vi "Leakdaten laden_speichern.vi"(6 "Aktion":T4(ring), 8 "error in (no error)":errorcluster caption="Fehler (Eingang, kein Fehler)", 9 "Leak Protokoll":T1={"Bearbeiter:"="", "Pfad:"=path "D:/IAG_Data/Log", "Textname:"="", "Analysator"=""} caption="T90 Konfig Daten", 11 "Gesamtvolumen":T3 {"LeakValve" items=["inactive", "active"]}) -> (0 "error out":errorcluster caption="Fehler (Ausgang)", 1 "Leak Protokoll":T1={"Bearbeiter:"="", "Pfad:"=path "D:/IAG_Data/Log", "Textname:"="", "Analysator"=""} caption="T90 Konfig Daten", 3 "Gesamtvolumen":T3 {"LeakValve" items=["inactive", "active"]})   [LabVIEW 2020, in "EPA 1065.lvlib" / "Dichtheitstest 1065-345.lvlib"]
uses:
  Dichtheitstest 1065-345.lvlib
  Gesamtvolumen.ctl
  Leak Protokoll Einstellungen.ctl
  Seiten/System Einstellungen V2/Analysatoren.ctl
  <vilib>/Utility/config.llb/Read Key (Double).vi
  <vilib>/Utility/config.llb/Read Key (Boolean).vi
  <vilib>/Utility/config.llb/Read Key (U32).vi
  <vilib>/Utility/config.llb/Write Key (Double).vi
  <vilib>/Utility/config.llb/Write Key (Boolean).vi
  <vilib>/Utility/config.llb/Write Key (U32).vi
  <vilib>/Utility/config.llb/Read Key (Path).vi
  <vilib>/Utility/config.llb/Read Key (String).vi
  <vilib>/Utility/config.llb/Write Key (Path).vi
  <vilib>/Utility/config.llb/Write Key (String).vi
  <vilib>/Utility/config.llb/NI_LVConfig.lvlib
  Allgemein/allgemeine Sub-VIs.lvlib
  Seiten/System Einstellungen V2/System Einstellungen V2.lvlib
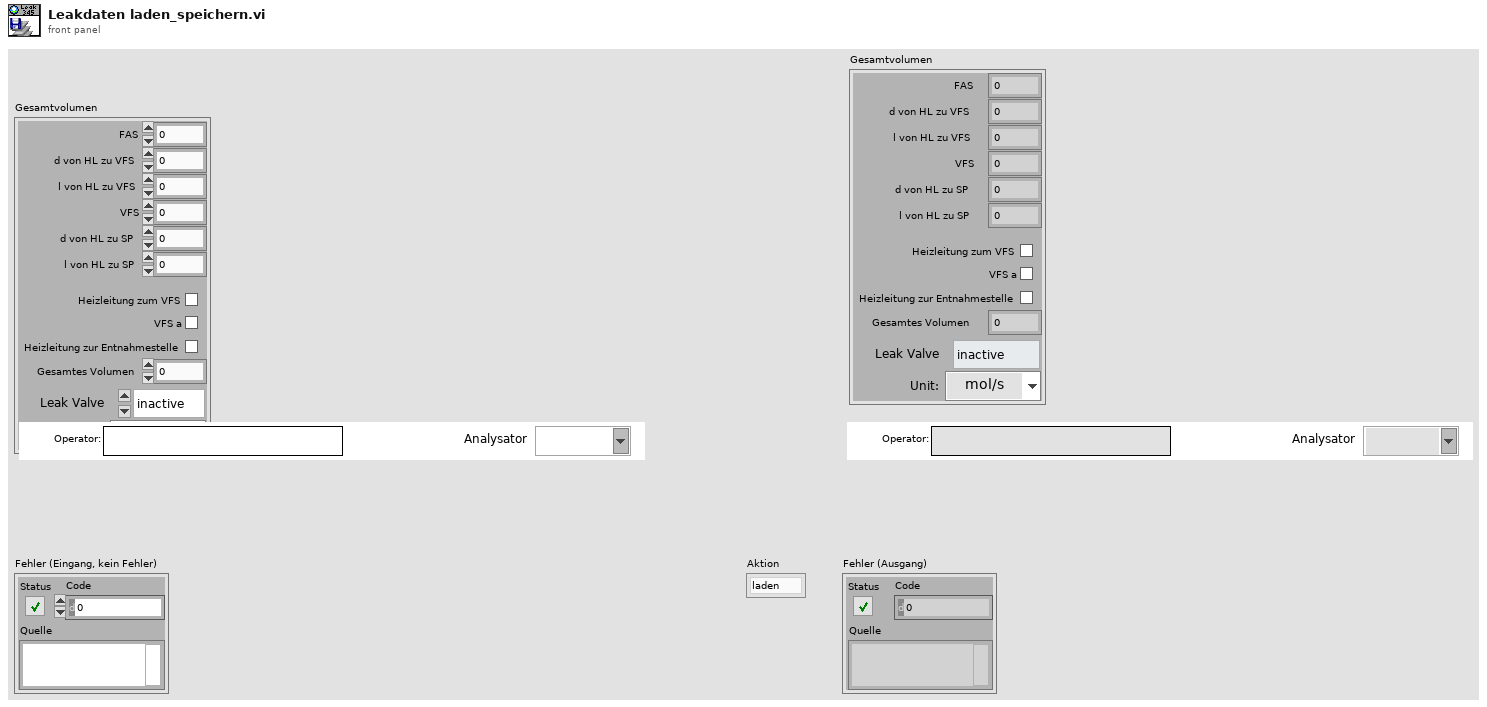
[diagram p1: front panel]
types:
  T1 = typedef "EPA 1065.lvlib/Dichtheitstest 1065-345.lvlib/Leak Protokoll Einstellungen.ctl" = cluster{"Bearbeiter:":string, "Pfad:":path, "Textname:":string, "Analysator":T2}
  T2 = typedef "System Einstellungen V2.lvlib/Analysatoren.ctl" = string
  T3 = typedef "EPA 1065.lvlib/Dichtheitstest 1065-345.lvlib/Gesamtvolumen.ctl" = cluster{"FAS":sgl, "d von HL zu VFS":sgl, "l von HL zu VFS":sgl, "VFS":sgl, "d von HL zu SP":sgl, "l von HL zu SP":sgl, "Heizleitung zum VFS":bool, "VFS a":bool, "Heizleitung zur Entnahmestelle":bool, "Gesamtes Volumen":sgl, "LeakValve":u16, "Einheit":enum16{"mol/s", "mbar"}}
  T4 = enum16{"laden", "speichern", "Pfad laden", "Pfad speichern"}
  T5 = typedef "NI_LVConfig.lvlib/Config Data RefNum.ctl" = refnum<k1>
  T6 = cluster{sgl, sgl, sgl, sgl, sgl, sgl, "value":bool, "value":bool, "value":bool, sgl, u16, u16}
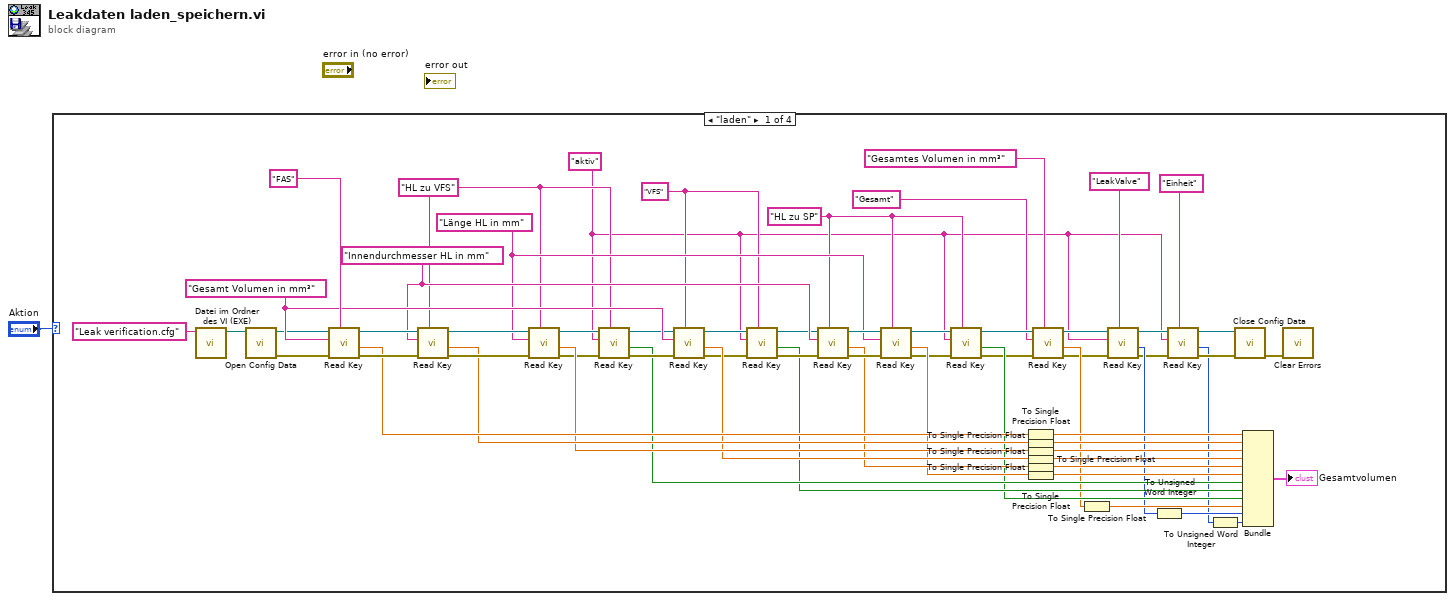
[diagram p0: block diagram]
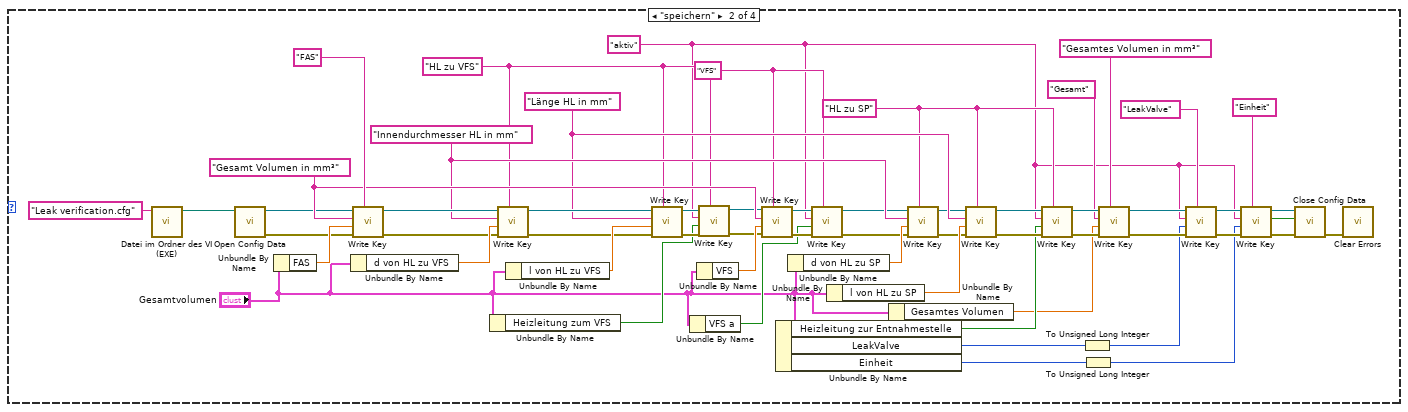
[diagram p2: hidden frame]
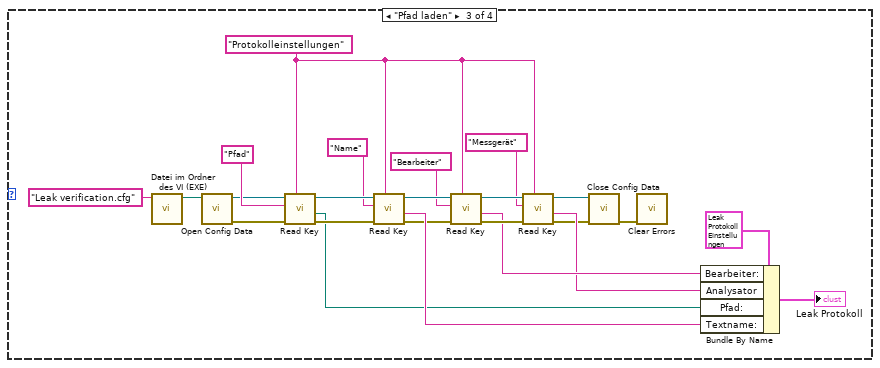
[diagram p3: hidden frame]
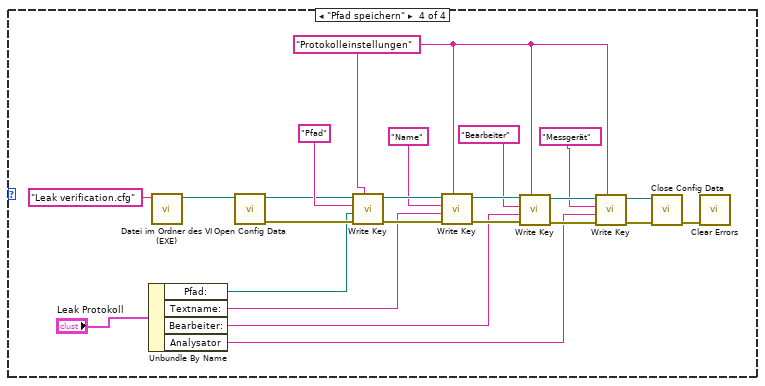
[diagram p4: hidden frame]
diagram:
  n1 = case shown="\"laden\"" "Aktion" {
    frame "laden" {
      w4 = "aktiv" ("key")
      w33 = "VFS"
      w29 = "HL zu SP"
      w55 = "Länge HL in mm" ("key")
      w56 = "Innendurchmesser HL in mm" ("key")
      w41 = "HL zu VFS"
      w57 = "Gesamt Volumen in mm³" ("key")
      n2 = call "Datei im Ordner des VI (EXE).vi"("Dateiname"="Leak verification.cfg") -> ("Dateipfad im Ordner des Haupt-VIs"=w51:path)  [unwired: 8 in, 2 out]
      n3 = call <vilib>:"Open Config Data.vi"("configuration file path"=w51) -> ("error out"=w53:errorcluster, "refnum"=w52:T5)  [unwired: 8 in, 1 out]
      n4 = call-poly <vilib>:"Read Key.vi"("section"="FAS", "error in (no error)"=w53, "key"=w57, "refnum"=w52) -> ("error out"=w61:errorcluster, "value"=w49:dbl, "refnum out"=w62:T5)  [unwired: 4 in, 1 out]
      n5 = call-poly <vilib>:"Read Key.vi"("section"=w41, "error in (no error)"=w61, "key"=w56, "refnum"=w62) -> ("error out"=w59:errorcluster, "value"=w48:dbl, "refnum out"=w63:T5)  [unwired: 4 in, 1 out]
      n6 = call-poly <vilib>:"Read Key.vi"("section"=w41, "error in (no error)"=w59, "key"=w55, "refnum"=w63) -> ("error out"=w40:errorcluster, "value"=w47:dbl, "refnum out"=w43:T5)  [unwired: 4 in, 1 out]
      n7 = call-poly <vilib>:"Read Key.vi"("section"=w41, "error in (no error)"=w40, "key"=w4, "refnum"=w43) -> ("error out"=w39:errorcluster, "value"=w38:bool, "refnum out"=w42:T5)  [unwired: 4 in, 1 out]
      n8 = call-poly <vilib>:"Read Key.vi"("section"=w33, "error in (no error)"=w39, "key"=w57, "refnum"=w42) -> ("error out"=w36:errorcluster, "value"=w46:dbl, "refnum out"=w37:T5)  [unwired: 4 in, 1 out]
      n9 = call-poly <vilib>:"Read Key.vi"("section"=w33, "error in (no error)"=w36, "key"=w4, "refnum"=w37) -> ("error out"=w35:errorcluster, "value"=w32:bool, "refnum out"=w34:T5)  [unwired: 4 in, 1 out]
      n10 = call-poly <vilib>:"Read Key.vi"("section"=w29, "error in (no error)"=w35, "key"=w56, "refnum"=w34) -> ("error out"=w58:errorcluster, "value"=w45:dbl, "refnum out"=w60:T5)  [unwired: 4 in, 1 out]
      n11 = call-poly <vilib>:"Read Key.vi"("section"=w29, "error in (no error)"=w58, "key"=w55, "refnum"=w60) -> ("error out"=w30:errorcluster, "value"=w44:dbl, "refnum out"=w31:T5)  [unwired: 4 in, 1 out]
      n12 = call-poly <vilib>:"Read Key.vi"("section"=w29, "error in (no error)"=w30, "key"=w4, "refnum"=w31) -> ("error out"=w19:errorcluster, "value"=w28:bool, "refnum out"=w18:T5)  [unwired: 4 in, 1 out]
      n13 = To Single Precision Float(number=w49) -> (single precision float=w26:sgl)
      n14 = To Single Precision Float(number=w48) -> (single precision float=w25:sgl)
      n15 = To Single Precision Float(number=w47) -> (single precision float=w24:sgl)
      n16 = To Single Precision Float(number=w46) -> (single precision float=w23:sgl)
      n17 = To Single Precision Float(number=w45) -> (single precision float=w22:sgl)
      n18 = To Single Precision Float(number=w44) -> (single precision float=w21:sgl)
      n19 = call-poly <vilib>:"Read Key.vi"("section"="Gesamtes Volumen in mm³", "error in (no error)"=w19, "key"="Gesamt", "refnum"=w18) -> ("error out"=w13:errorcluster, "value"=w17:dbl, "refnum out"=w14:T5)  [unwired: 4 in, 1 out]
      n20 = To Single Precision Float(number=w17) -> (single precision float=w20:sgl)
      n21 = call-poly <vilib>:"Read Key.vi"("section"="LeakValve", "error in (no error)"=w13, "key"=w4, "refnum"=w14) -> ("error out"=w9:errorcluster, "value"=w10:u32, "refnum out"=w8:T5)  [unwired: 4 in, 1 out]
      n22 = To Unsigned Word Integer(number=w10) -> (unsigned 16bit integer=w11:u16)
      n23 = call-poly <vilib>:"Read Key.vi"("section"="Einheit" ("key"), "error in (no error)"=w9, "key"=w4, "refnum"=w8) -> ("error out"=w6:errorcluster, "value"=w3:u32, "refnum out"=w7:T5)  [unwired: 4 in, 1 out]
      n24 = To Unsigned Word Integer(number=w3) -> (unsigned 16bit integer=w2:u16)
      n25 = call <vilib>:"Close Config Data.vi"("error in (no error)"=w6, "refnum"=w7) -> ("error out"=w54:errorcluster)  [unwired: 8 in, 1 out]
      n26 = Bundle(w26, w25, w24, w23, w22, w21, "value"=w38, "value"=w32, "value"=w28, w20, w11, w2) -> (→"Gesamtvolumen":T6)  [unwired: 1 in]
      n27 = call <vilib>:"Clear Errors.vi"("error in (no error)"=w54) -> ()  [unwired: 5 in, 2 out]
    }
    frame "speichern" {
      w69 = "aktiv" ("key")
      w92 = "VFS"
      w86 = "HL zu SP"
      w108 = "Länge HL in mm" ("key")
      w109 = "Innendurchmesser HL in mm" ("key")
      w97 = "HL zu VFS"
      w110 = "Gesamt Volumen in mm³" ("key")
      n28 = call "Datei im Ordner des VI (EXE).vi"("Dateiname"="Leak verification.cfg") -> ("Dateipfad im Ordner des Haupt-VIs"=w104:path)  [unwired: 8 in, 2 out]
      n29 = call <vilib>:"Open Config Data.vi"("configuration file path"=w104) -> ("error out"=w106:errorcluster, "refnum"=w105:T5)  [unwired: 8 in, 1 out]
      n30 = Unbundle By Name("Gesamtvolumen") -> ("FAS"=w120:sgl)
      n31 = Unbundle By Name("Gesamtvolumen") -> ("d von HL zu VFS"=w119:sgl)
      n32 = call-poly <vilib>:"Write Key.vi"("section"="FAS", "error in (no error)"=w106, "value"=w120, "key"=w110, "refnum"=w105) -> ("error out"=w115:errorcluster, "refnum out"=w116:T5)  [unwired: 4 in, 1 out]
      n33 = Unbundle By Name("Gesamtvolumen") -> ("Heizleitung zum VFS"=w98:bool)
      n34 = call-poly <vilib>:"Write Key.vi"("section"=w97, "error in (no error)"=w115, "value"=w119, "key"=w109, "refnum"=w116) -> ("error out"=w111:errorcluster, "refnum out"=w117:T5)  [unwired: 4 in, 1 out]
      n35 = Unbundle By Name("Gesamtvolumen") -> ("l von HL zu VFS"=w118:sgl)
      n36 = call-poly <vilib>:"Write Key.vi"("section"=w97, "error in (no error)"=w111, "value"=w118, "key"=w108, "refnum"=w117) -> ("error out"=w102:errorcluster, "refnum out"=w101:T5)  [unwired: 4 in, 1 out]
      n37 = Unbundle By Name("Gesamtvolumen") -> ("VFS a"=w91:bool)
      n38 = Unbundle By Name("Gesamtvolumen") -> ("VFS"=w112:sgl)
      n39 = call-poly <vilib>:"Write Key.vi"("section"=w97, "error in (no error)"=w102, "value"=w98, "key"=w69, "refnum"=w101) -> ("error out"=w99:errorcluster, "refnum out"=w100:T5)  [unwired: 4 in, 1 out]
      n40 = call-poly <vilib>:"Write Key.vi"("section"=w92, "error in (no error)"=w99, "value"=w112, "key"=w110, "refnum"=w100) -> ("error out"=w96:errorcluster, "refnum out"=w95:T5)  [unwired: 4 in, 1 out]
      n41 = Unbundle By Name("Gesamtvolumen") -> ("Heizleitung zur Entnahmestelle"=w85:bool, "LeakValve"=w68:u16, "Einheit"=w66:enum16{"mol/s", "mbar"})
      n42 = Unbundle By Name("Gesamtvolumen") -> ("d von HL zu SP"=w113:sgl)
      n43 = call-poly <vilib>:"Write Key.vi"("section"=w92, "error in (no error)"=w96, "value"=w91, "key"=w69, "refnum"=w95) -> ("error out"=w93:errorcluster, "refnum out"=w94:T5)  [unwired: 4 in, 1 out]
      n44 = Unbundle By Name("Gesamtvolumen") -> ("l von HL zu SP"=w114:sgl)
      n45 = Unbundle By Name("Gesamtvolumen") -> ("Gesamtes Volumen"=w79:sgl)
      n46 = call-poly <vilib>:"Write Key.vi"("section"=w86, "error in (no error)"=w93, "value"=w113, "key"=w109, "refnum"=w94) -> ("error out"=w89:errorcluster, "refnum out"=w90:T5)  [unwired: 4 in, 1 out]
      n47 = call-poly <vilib>:"Write Key.vi"("section"=w86, "error in (no error)"=w89, "value"=w114, "key"=w108, "refnum"=w90) -> ("error out"=w88:errorcluster, "refnum out"=w87:T5)  [unwired: 4 in, 1 out]
      n48 = call-poly <vilib>:"Write Key.vi"("section"=w86, "error in (no error)"=w88, "value"=w85, "key"=w69, "refnum"=w87) -> ("error out"=w84:errorcluster, "refnum out"=w83:T5)  [unwired: 4 in, 1 out]
      n49 = To Unsigned Long Integer(number=w68) -> (unsigned 32bit integer=w67:u32)
      n50 = To Unsigned Long Integer(number=w66) -> (unsigned 32bit integer=w65:u32)
      n51 = call-poly <vilib>:"Write Key.vi"("section"="Gesamtes Volumen in mm³", "error in (no error)"=w84, "value"=w79, "key"="Gesamt", "refnum"=w83) -> ("error out"=w73:errorcluster, "refnum out"=w78:T5)  [unwired: 4 in, 1 out]
      n52 = call-poly <vilib>:"Write Key.vi"("section"="LeakValve", "error in (no error)"=w73, "value"=w67, "key"=w69, "refnum"=w78) -> ("error out"=w72:errorcluster, "refnum out"=w75:T5)  [unwired: 4 in, 1 out]
      n53 = call-poly <vilib>:"Write Key.vi"("section"="Einheit", "error in (no error)"=w72, "value"=w65, "key"=w69, "refnum"=w75) -> ("error out"=w71:errorcluster, "found?"=w76:bool, "refnum out"=w74:T5)  [unwired: 4 in]
      n54 = call <vilib>:"Close Config Data.vi"("error in (no error)"=w71, "write file if changed (T)"=w76, "refnum"=w74) -> ("error out"=w107:errorcluster)  [unwired: 7 in, 1 out]
      n55 = call <vilib>:"Clear Errors.vi"("error in (no error)"=w107) -> ()  [unwired: 5 in, 2 out]
    }
    frame "Pfad laden" {
      w126 = "Protokolleinstellungen"
      n56 = call "Datei im Ordner des VI (EXE).vi"("Dateiname"="Leak verification.cfg") -> ("Dateipfad im Ordner des Haupt-VIs"=w138:path)  [unwired: 8 in, 2 out]
      n57 = call <vilib>:"Open Config Data.vi"("configuration file path"=w138) -> ("error out"=w140:errorcluster, "refnum"=w139:T5)  [unwired: 8 in, 1 out]
      n58 = call-poly <vilib>:"Read Key.vi"("section"=w126, "error in (no error)"=w140, "key"="Pfad", "refnum"=w139) -> ("error out"=w144:errorcluster, "value"=w134:path, "refnum out"=w145:T5)  [unwired: 4 in, 1 out]
      n59 = call-poly <vilib>:"Read Key.vi"("section"=w126, "error in (no error)"=w144, "key"="Name", "refnum"=w145) -> ("error out"=w131:errorcluster, "value"=w135:string, "refnum out"=w132:T5)  [unwired: 4 in, 1 out]
      n60 = call-poly <vilib>:"Read Key.vi"("section"=w126, "error in (no error)"=w131, "key"="Bearbeiter", "refnum"=w132) -> ("error out"=w130:errorcluster, "value"=w125:string, "refnum out"=w129:T5)  [unwired: 4 in, 1 out]
      n61 = call-poly <vilib>:"Read Key.vi"("section"=w126, "error in (no error)"=w130, "key"="Messgerät", "refnum"=w129) -> ("error out"=w123:errorcluster, "value"=w124:string, "refnum out"=w122:T5)  [unwired: 4 in, 1 out]
      n62 = call <vilib>:"Close Config Data.vi"("error in (no error)"=w123, "refnum"=w122) -> ("error out"=w141:errorcluster)  [unwired: 8 in, 1 out]
      n63 = call <vilib>:"Clear Errors.vi"("error in (no error)"=w141) -> ()  [unwired: 5 in, 2 out]
      n64 = Bundle By Name(cluster=T1 {"Bearbeiter:"="", "Pfad:"=path "D:/IAG_Data/Log", "Textname:"="", "Analysator"=""} ("Leak Protokoll"), "Bearbeiter:"=w125, "Analysator"=w124, "Pfad:"=w134, "Textname:"=w135) -> (→"Leak Protokoll":T1)
    }
    frame "Pfad speichern" {
      w147 = "Protokolleinstellungen"
      n65 = Unbundle By Name("Leak Protokoll") -> ("Pfad:"=w158:path, "Textname:"=w157:string, "Bearbeiter:"=w152:string, "Analysator"=w146:T2)
      n66 = call "Datei im Ordner des VI (EXE).vi"("Dateiname"="Leak verification.cfg") -> ("Dateipfad im Ordner des Haupt-VIs"=w161:path)  [unwired: 8 in, 2 out]
      n67 = call <vilib>:"Open Config Data.vi"("configuration file path"=w161) -> ("error out"=w163:errorcluster, "refnum"=w162:T5)  [unwired: 8 in, 1 out]
      n68 = call-poly <vilib>:"Write Key.vi"("section"=w147, "error in (no error)"=w163, "value"=w158, "key"="Pfad", "refnum"=w162) -> ("error out"=w167:errorcluster, "refnum out"=w168:T5)  [unwired: 4 in, 1 out]
      n69 = call-poly <vilib>:"Write Key.vi"("section"=w147, "error in (no error)"=w167, "value"=w157, "key"="Name", "refnum"=w168) -> ("error out"=w155:errorcluster, "refnum out"=w156:T5)  [unwired: 4 in, 1 out]
      n70 = call-poly <vilib>:"Write Key.vi"("section"=w147, "error in (no error)"=w155, "value"=w152, "key"="Bearbeiter", "refnum"=w156) -> ("error out"=w151:errorcluster, "refnum out"=w153:T5)  [unwired: 4 in, 1 out]
      n71 = call-poly <vilib>:"Write Key.vi"("section"=w147, "error in (no error)"=w151, "value"=w146, "key"="Messgerät", "refnum"=w153) -> ("error out"=w148:errorcluster, "refnum out"=w149:T5)  [unwired: 4 in, 1 out]
      n72 = call <vilib>:"Close Config Data.vi"("error in (no error)"=w148, "refnum"=w149) -> ("error out"=w164:errorcluster)  [unwired: 8 in, 1 out]
      n73 = call <vilib>:"Clear Errors.vi"("error in (no error)"=w164) -> ()  [unwired: 5 in, 2 out]
    }
  }
